vi "20.1.E122X.Group4.FinalExperimentAnalysis.vi"() -> ()   [LabVIEW 2014]
uses:
  <vilib>/Utility/miscctls.llb/LVDateTimeRec.ctl
  <vilib>/Analysis/baseanly.llb/Mean (DBL).vi
  <vilib>/Utility/file.llb/Read From Spreadsheet File (string).vi
  <vilib>/regexp/Match Regular Expression.xnode
  <vilib>/Analysis/NI_AALBase.lvlib
panel:
  in  "file path: CPU/GPU":path
  in  "file path: Environment":path
  in  "Tab Control":T1(tab)
  out "GPU":cluster{timestamp[], dbl[]}(graph)
  out "CPU":cluster{timestamp[], dbl[]}(graph)
  out "Humidity":cluster{timestamp[], dbl[]}(graph)
  out "Temperature":cluster{timestamp[], dbl[]}(graph)
  in  "Window Position":dbl(slide) min=3670814882.0 max=3671117162.0 scale=3670814882.0..3671117162.0 scale format="%<%I:%M %p\n%m/%d>T"
  in  "Window Size":dbl(slide) min=3670814882.0 max=3671117162.0 scale=240.0..302280.0 scale format="%<%H:%M>t"
  out "Light":cluster{timestamp[], dbl[]}(graph)
  out "Current Time":dbl format="%<%X\n%x>T"
  out "Light at index":dbl
  out "Humidity at index":dbl
  out "Temperature at index":dbl
  out "Light Max":dbl
  out "Humidity Max":dbl
  out "Temperature Max":dbl
  out "Light Min":dbl
  out "Humidity Min":dbl
  out "Temperature Min":dbl
  out "Light Average":dbl
  out "Humidity Average":dbl
  out "Temperature Average":dbl
  in  "Data Index":i64(slide) scale=0.0..2146.0
  out "Low Sun (1200-5000 lux)":bool
  out "Overcast day (700-1200 lux)":bool
  out "Bright room (50-700 lux)":bool
  out "Dark room (5-50 lux)":bool
  out "Moonlit night (.5-5 lux)":bool
  out "Dim Hallway (.01-.1 lux)":bool
  # "This section contains information to verify that the system is functional."
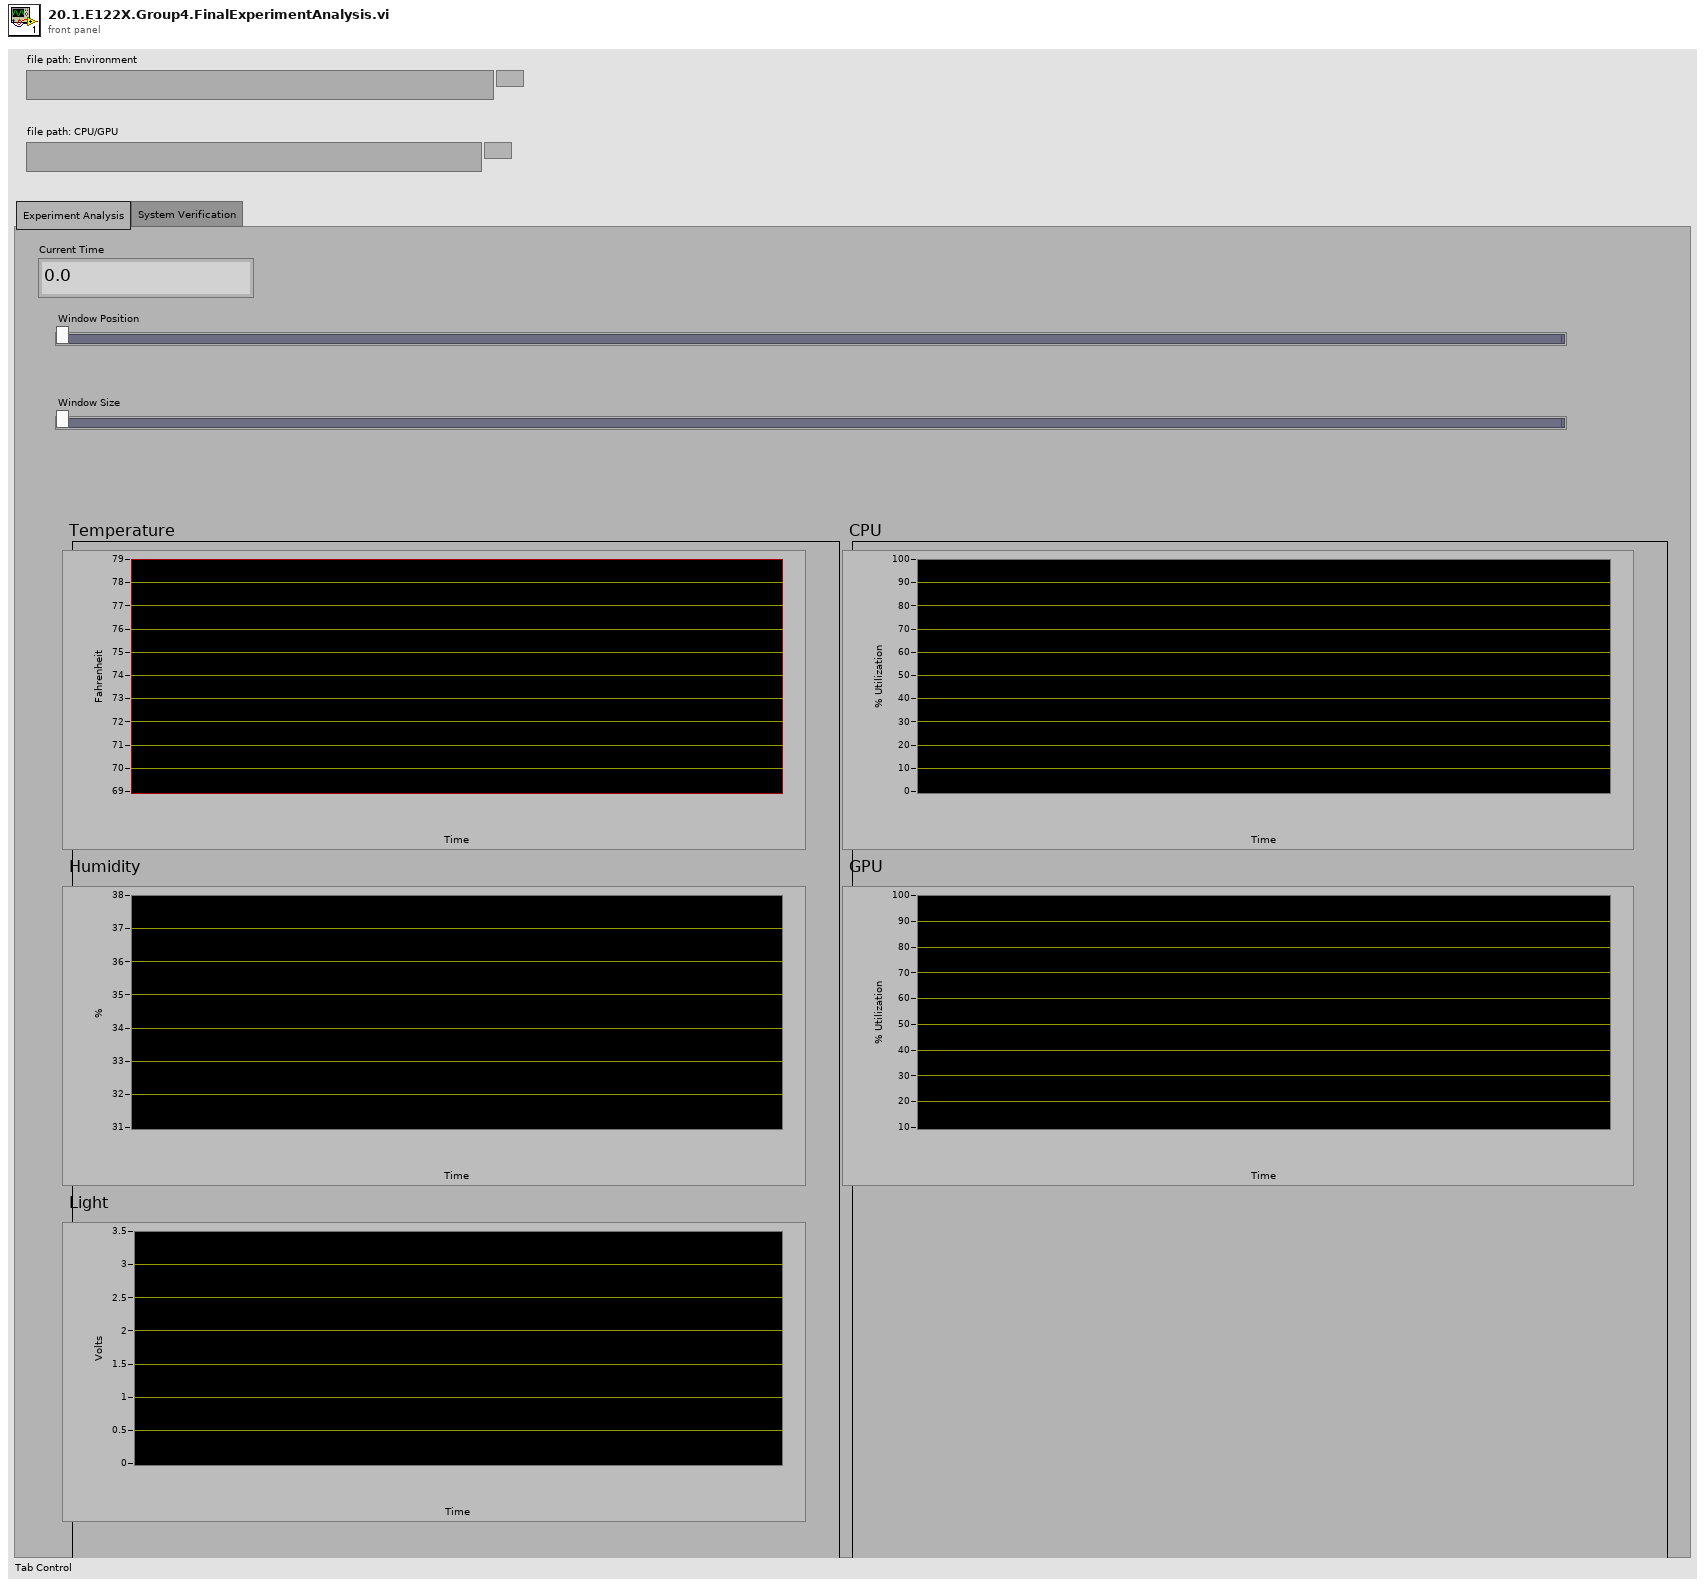
[diagram p1: front panel]
types:
  T1 = enum32{"Experiment Analysis", "System Verification"}
  T2 = typedef "LVDateTimeRec.ctl" = cluster{"fractional second":dbl, "second":i32, "minute":i32, "hour":i32, "day of month":i32, "month":i32, "year":i32, "day of week":i32, "day of year":i32, "DST":i32}
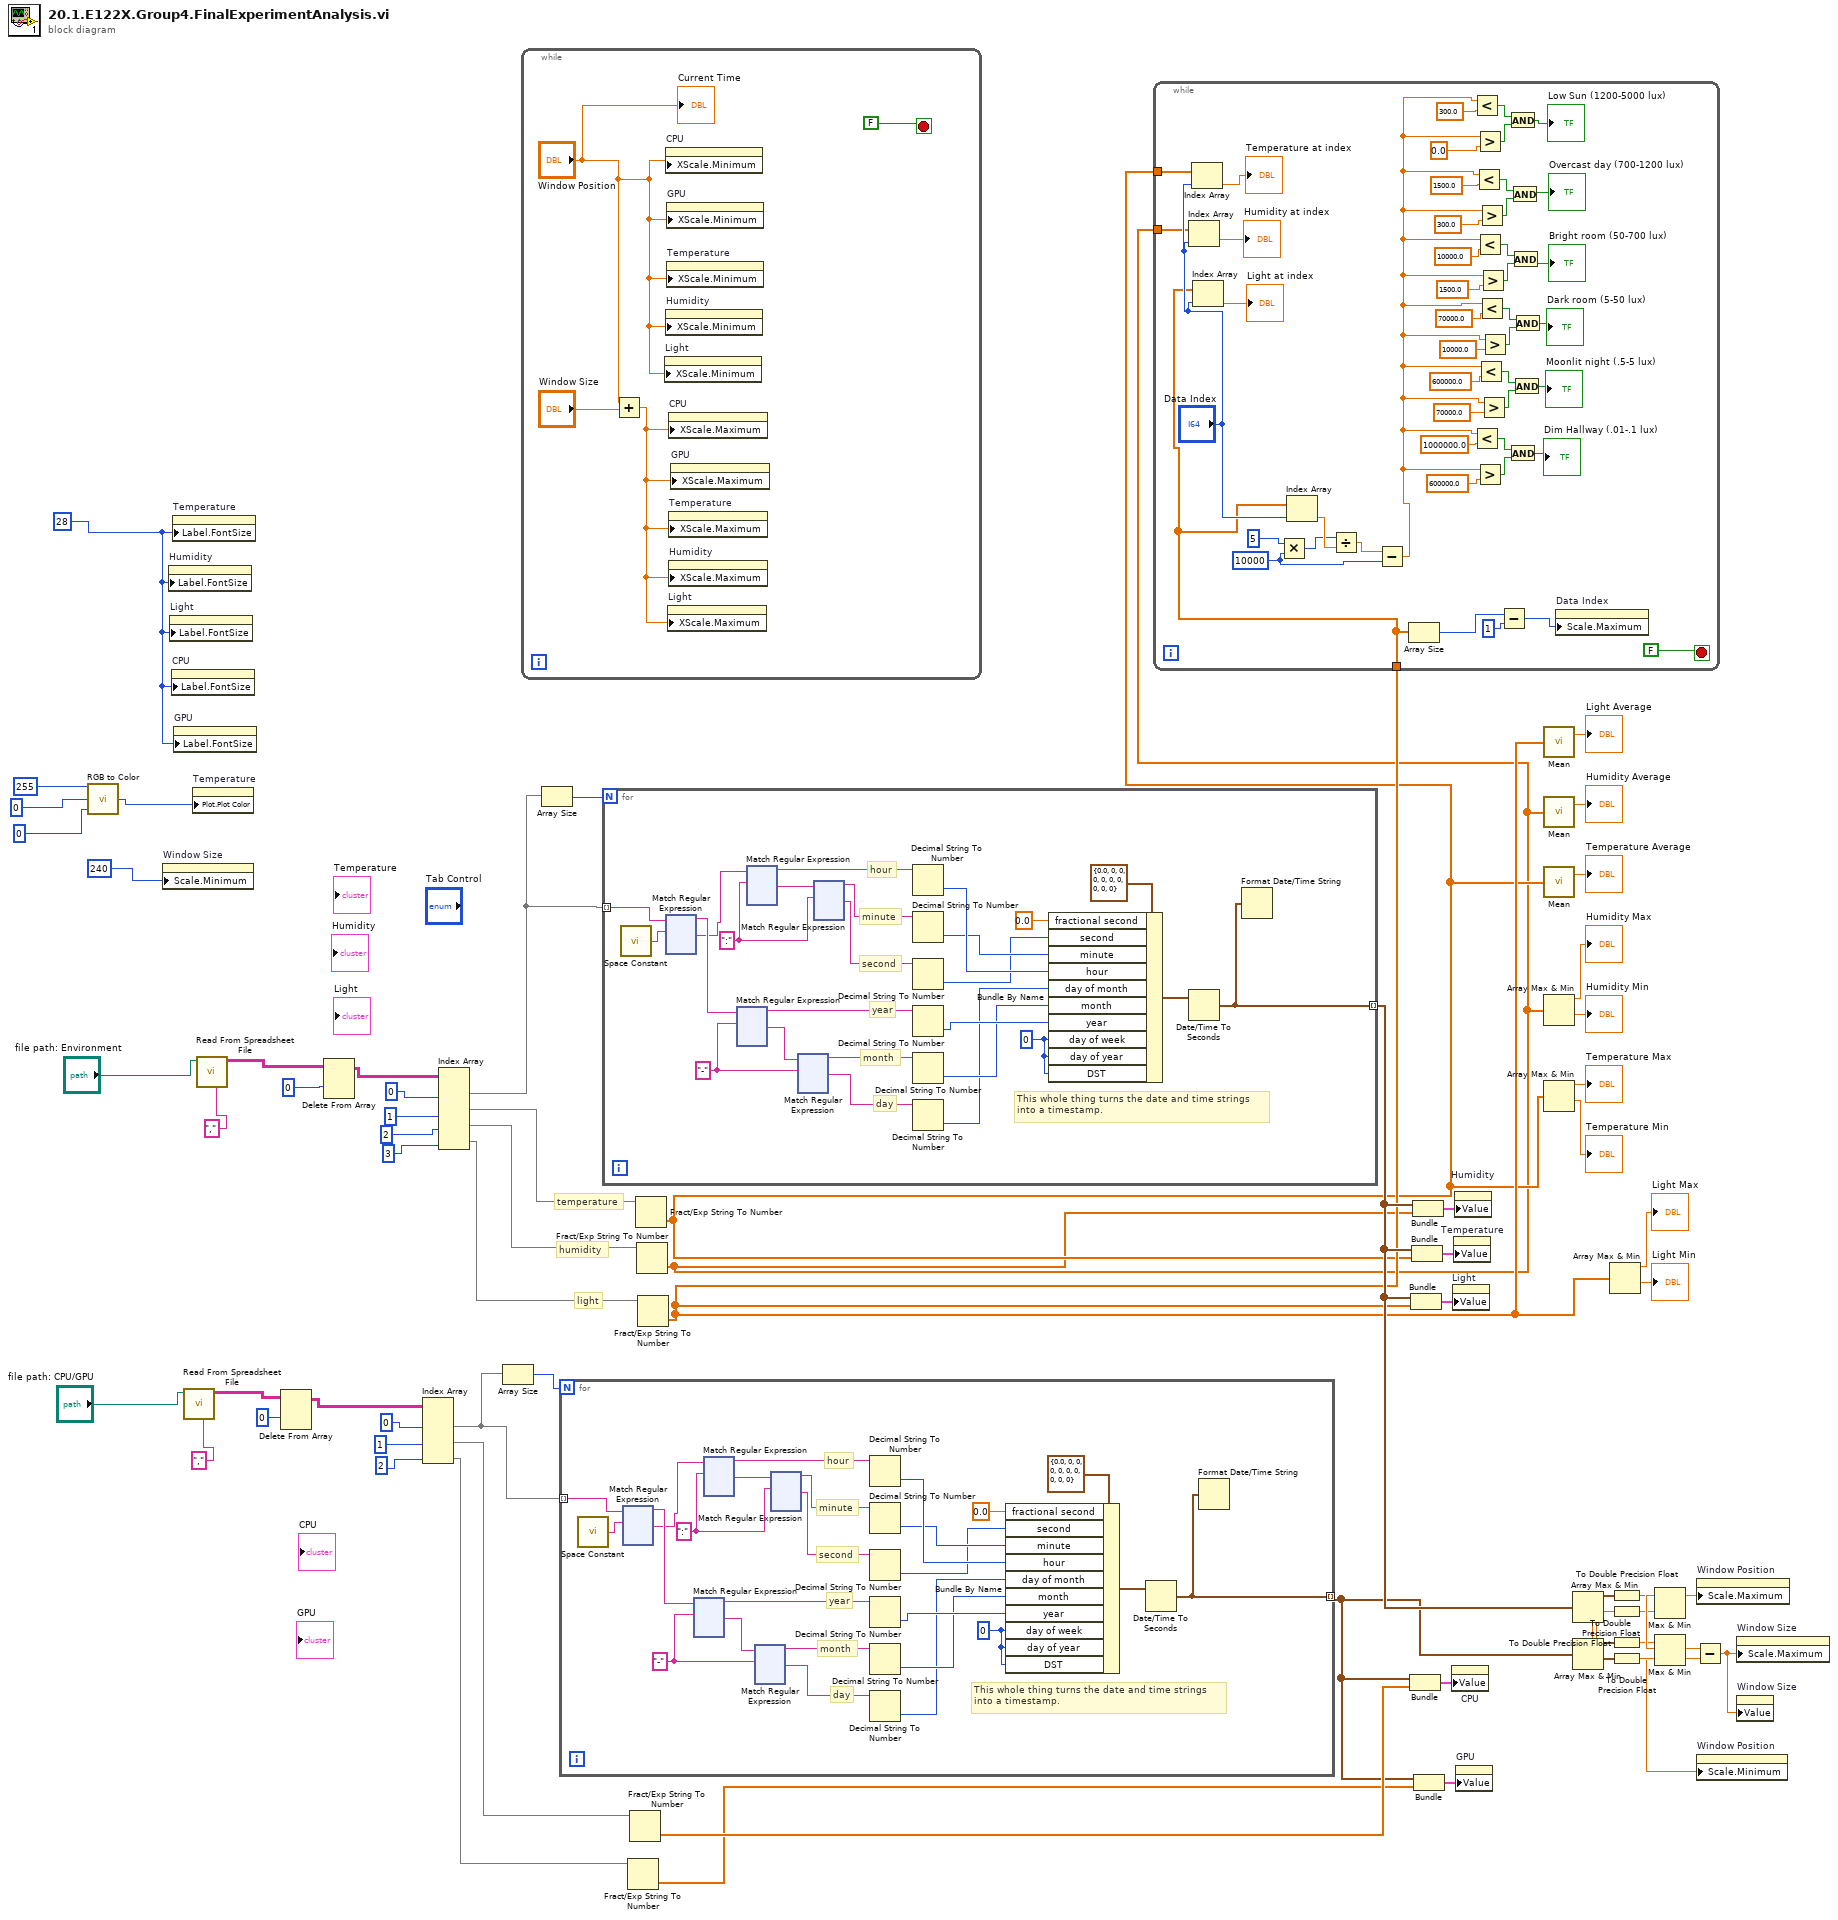
[diagram p0: block diagram]
diagram:
  w14 = 28
  # "light"
  # "humidity"
  # "temperature"
  n1 = call <vilib>:"RGB to Color.vi"("B"=0, "G"=0, "R"=255) -> ("Color"=w18:u32)
  n2 = property on="Window Size" class="Slide (strict)"("Scale.Minimum"=240) -> ()  [unwired: 2 in, 2 out]
  n3 = property on="Humidity" class="XYGraph (strict)"("Label.FontSize"=w14) -> ()  [unwired: 2 in, 2 out]
  n4 = property on="Light" class="XYGraph (strict)"("Label.FontSize"=w14) -> ()  [unwired: 2 in, 2 out]
  n5 = property on="CPU" class="XYGraph (strict)"("Label.FontSize"=w14) -> ()  [unwired: 2 in, 2 out]
  n6 = property on="Temperature" class="XYGraph (strict)"("Label.FontSize"=w14) -> ()  [unwired: 2 in, 2 out]
  n7 = property on="GPU" class="XYGraph (strict)"("Label.FontSize"=w14) -> ()  [unwired: 2 in, 2 out]
  n8 = call-poly <vilib>:"Read From Spreadsheet File.vi"("delimiter (\\t)"="," ("delimiter (\\t)"), "file path (dialog if empty)"="file path: CPU/GPU") -> ("all rows"=w54:string[][])  [unwired: 5 in, 4 out]
  n9 = property on="Temperature" class="XYGraph (strict)"("Plot.Plot Color"=w18) -> ()  [unwired: 2 in, 2 out]
  n10 = call-poly <vilib>:"Read From Spreadsheet File.vi"("delimiter (\\t)"="," ("delimiter (\\t)"), "file path (dialog if empty)"="file path: Environment") -> ("all rows"=w56:string[][])  [unwired: 5 in, 4 out]
  n11 = Delete From Array(array=w54, index (row)=0) -> (array with subset deleted=w46:string[][])  [unwired: 2 in, 1 out]
  n12 = Delete From Array(array=w56, index (row)=0) -> (array with subset deleted=w52:string[][])  [unwired: 2 in, 1 out]
  n13 = Index Array(array=w46, index (col) #1=0 ("disabled index (col)"), index (col) #2=1 ("disabled index (col)"), index (col) #3=2 ("disabled index (col)")) -> (element #1=w42:string[], element #2=w44:string[], element #3=w45:string[])  [unwired: 3 in]
  n14 = Index Array(array=w52, index (col) #1=0 ("disabled index (col)"), index (col) #2=1 ("index (col)"), index (col) #3=2 ("index (col)"), index (col) #4=3 ("index (col)")) -> (element #1=w50:string[], element #2=w49:string[], element #3=w48:string[], element #4=w47:string[])  [unwired: 4 in]
  n15 = Array Size(array=w42) -> (size(s)=w43:i32)
  n16 = while {
    stop <- FALSE stop-if-true
    n17 = Add(x="Window Position", y="Window Size") -> (x+y=w65:dbl)
    n18 = property on="Light" class="XYGraph (strict)"("XScale.Minimum"="Window Position") -> ()  [unwired: 2 in, 2 out]
    n19 = property on="CPU" class="XYGraph (strict)"("XScale.Minimum"="Window Position") -> ()  [unwired: 2 in, 2 out]
    n20 = property on="Humidity" class="XYGraph (strict)"("XScale.Minimum"="Window Position") -> ()  [unwired: 2 in, 2 out]
    n21 = property on="GPU" class="XYGraph (strict)"("XScale.Minimum"="Window Position") -> ()  [unwired: 2 in, 2 out]
    n22 = property on="Temperature" class="XYGraph (strict)"("XScale.Minimum"="Window Position") -> ()  [unwired: 2 in, 2 out]
    n23 = property on="Light" class="XYGraph (strict)"("XScale.Maximum"=w65) -> ()  [unwired: 2 in, 2 out]
    n24 = property on="CPU" class="XYGraph (strict)"("XScale.Maximum"=w65) -> ()  [unwired: 2 in, 2 out]
    n25 = property on="Temperature" class="XYGraph (strict)"("XScale.Maximum"=w65) -> ()  [unwired: 2 in, 2 out]
    n26 = property on="Humidity" class="XYGraph (strict)"("XScale.Maximum"=w65) -> ()  [unwired: 2 in, 2 out]
    n27 = property on="GPU" class="XYGraph (strict)"("XScale.Maximum"=w65) -> ()  [unwired: 2 in, 2 out]
    "Current Time" <- "Window Position"
  }
  n28 = Array Size(array=w50) -> (size(s)=w51:i32)
  n29 = for {
    N: w43 -> [_]
    tunnel: w42 -> [w75] mode=indexing
    tunnel: [w69] -> w13 mode=indexing
    w79 = 0 ("day of week")
    w76 = ":" ("regular expression")
    w93 = "-" ("regular expression")
    # "This whole thing turns the date and time strings\ninto a timestamp."
    # "second"
    # "minute"
    # "hour"
    # "year"
    # "day"
    # "month"
    n30 = call <vilib>:"Space Constant.vi"() -> ("String"=w77:string)
    n31 = xnode "Match Regular Expression"("input string"=w75, "regular expression"=w77) -> ("before match"=w71:string, "after match"=w70:string)  [unwired: 4 in, 3 out]
    n32 = xnode "Match Regular Expression"("input string"=w71, "regular expression"=w93) -> ("before match"=w90:string, "after match"=w92:string)  [unwired: 4 in, 3 out]
    n33 = xnode "Match Regular Expression"("input string"=w70, "regular expression"=w76) -> ("before match"=w87:string, "after match"=w91:string)  [unwired: 4 in, 3 out]
    n34 = xnode "Match Regular Expression"("input string"=w92, "regular expression"=w93) -> ("before match"=w89:string, "after match"=w88:string)  [unwired: 4 in, 3 out]
    n35 = xnode "Match Regular Expression"("input string"=w91, "regular expression"=w76) -> ("before match"=w86:string, "after match"=w85:string)  [unwired: 4 in, 3 out]
    n36 = Decimal String To Number(string=w87) -> (number=w83:i32)  [unwired: 2 in, 1 out]
    n37 = Decimal String To Number(string=w86) -> (number=w82:i32)  [unwired: 2 in, 1 out]
    n38 = Decimal String To Number(string=w85) -> (number=w81:i32)  [unwired: 2 in, 1 out]
    n39 = Decimal String To Number(string=w90) -> (number=w74:i32)  [unwired: 2 in, 1 out]
    n40 = Decimal String To Number(string=w89) -> (number=w73:i32)  [unwired: 2 in, 1 out]
    n41 = Decimal String To Number(string=w88) -> (number=w72:i32)  [unwired: 2 in, 1 out]
    n42 = Bundle By Name(cluster=T2 {"fractional second"=0.0, "second"=0, "minute"=0, "hour"=0, "day of month"=0, "month"=0, "year"=0, "day of week"=0, "day of year"=0, "DST"=0} ("date time rec"), "fractional second"=0.0, "second"=w81, "minute"=w82, "hour"=w83, "day of month"=w72, "month"=w73, "year"=w74, "day of week"=w79, "day of year"=w79, "DST"=w79) -> (w80:T2)
    n43 = Date/Time To Seconds(2:w80) -> (0:w69:timestamp)  [unwired: 1 in]
    n44 = Format Date/Time String(seconds (now)=w69) -> ()  [unwired: 2 in, 1 out]
  }
  n45 = for {
    N: w51 -> [_]
    tunnel: w50 -> [w670] mode=indexing
    tunnel: [w664] -> w24 mode=indexing
    w674 = 0 ("day of week")
    w671 = ":" ("regular expression")
    w688 = "-" ("regular expression")
    # "This whole thing turns the date and time strings\ninto a timestamp."
    # "second"
    # "minute"
    # "hour"
    # "year"
    # "day"
    # "month"
    n46 = call <vilib>:"Space Constant.vi"() -> ("String"=w672:string)
    n47 = xnode "Match Regular Expression"("input string"=w670, "regular expression"=w672) -> ("before match"=w666:string, "after match"=w665:string)  [unwired: 4 in, 3 out]
    n48 = xnode "Match Regular Expression"("input string"=w666, "regular expression"=w688) -> ("before match"=w685:string, "after match"=w687:string)  [unwired: 4 in, 3 out]
    n49 = xnode "Match Regular Expression"("input string"=w665, "regular expression"=w671) -> ("before match"=w682:string, "after match"=w686:string)  [unwired: 4 in, 3 out]
    n50 = xnode "Match Regular Expression"("input string"=w687, "regular expression"=w688) -> ("before match"=w684:string, "after match"=w683:string)  [unwired: 4 in, 3 out]
    n51 = xnode "Match Regular Expression"("input string"=w686, "regular expression"=w671) -> ("before match"=w681:string, "after match"=w680:string)  [unwired: 4 in, 3 out]
    n52 = Decimal String To Number(string=w682) -> (number=w678:i32)  [unwired: 2 in, 1 out]
    n53 = Decimal String To Number(string=w681) -> (number=w677:i32)  [unwired: 2 in, 1 out]
    n54 = Decimal String To Number(string=w680) -> (number=w676:i32)  [unwired: 2 in, 1 out]
    n55 = Decimal String To Number(string=w685) -> (number=w669:i32)  [unwired: 2 in, 1 out]
    n56 = Decimal String To Number(string=w684) -> (number=w668:i32)  [unwired: 2 in, 1 out]
    n57 = Decimal String To Number(string=w683) -> (number=w667:i32)  [unwired: 2 in, 1 out]
    n58 = Bundle By Name(cluster=T2 {"fractional second"=0.0, "second"=0, "minute"=0, "hour"=0, "day of month"=0, "month"=0, "year"=0, "day of week"=0, "day of year"=0, "DST"=0} ("date time rec"), "fractional second"=0.0, "second"=w676, "minute"=w677, "hour"=w678, "day of month"=w667, "month"=w668, "year"=w669, "day of week"=w674, "day of year"=w674, "DST"=w674) -> (w675:T2)
    n59 = Date/Time To Seconds(2:w675) -> (0:w664:timestamp)  [unwired: 1 in]
    n60 = Format Date/Time String(seconds (now)=w664) -> ()  [unwired: 2 in, 1 out]
  }
  n61 = Fract/Exp String To Number(string=w45) -> (number=w36:dbl[])  [unwired: 3 in, 1 out]
  n62 = Fract/Exp String To Number(string=w44) -> (number=w38:dbl[])  [unwired: 3 in, 1 out]
  n63 = Fract/Exp String To Number(string=w49) -> (number=w2:dbl[])  [unwired: 3 in, 1 out]
  n64 = Fract/Exp String To Number(string=w48) -> (number=w1:dbl[])  [unwired: 3 in, 1 out]
  n65 = Fract/Exp String To Number(string=w47) -> (number=w3:dbl[])  [unwired: 3 in, 1 out]
  n66 = while {
    tunnel: w3 -> [w1259]
    tunnel: w2 -> [w1261]
    tunnel: w1 -> [w1260]
    stop <- FALSE stop-if-true
    w1269 = 10000
    n67 = Index Array(array=w1260, index="Data Index") -> (element=→"Humidity at index":dbl)
    n68 = Index Array(array=w1261, index="Data Index") -> (element=→"Temperature at index":dbl)
    n69 = Index Array(array=w1259, index="Data Index") -> (element=→"Light at index":dbl)
    n70 = Multiply(x=5, y=w1269) -> (x*y=w1271:i32)
    n71 = Index Array(array=w1259, index="Data Index") -> (element=w1272:dbl)
    n72 = Divide(x=w1271, y=w1272) -> (x/y=w1274:dbl)
    n73 = Subtract(x=w1274, y=w1269) -> (x-y=w1273:dbl)
    n74 = Array Size(array=w1259) -> (size(s)=w1268:i32)
    n75 = Less?(x=w1273, y=300.0) -> (x < y?=w1301:bool)
    n76 = Less?(x=w1273, y=1000000.0) -> (x < y?=w1277:bool)
    n77 = Less?(x=w1273, y=1500.0) -> (x < y?=w1296:bool)
    n78 = Greater?(x=w1273, y=0.0) -> (0:w1302:bool)
    n79 = Less?(x=w1273, y=10000.0) -> (x < y?=w1291:bool)
    n80 = Greater?(x=w1273, y=600000.0) -> (0:w1278:bool)
    n81 = Less?(x=w1273, y=600000.0) -> (x < y?=w1281:bool)
    n82 = Greater?(x=w1273, y=300.0) -> (0:w1297:bool)
    n83 = Less?(x=w1273, y=70000.0) -> (x < y?=w1285:bool)
    n84 = Greater?(x=w1273, y=1500.0) -> (0:w1292:bool)
    n85 = Greater?(x=w1273, y=70000.0) -> (0:w1282:bool)
    n86 = Greater?(x=w1273, y=10000.0) -> (0:w1286:bool)
    n87 = Subtract(x=w1268, y=1) -> (x-y=w1267:i32)
    n88 = And(x=w1301, y=w1302) -> (x .and. y?=→"Low Sun (1200-5000 lux)":bool)
    n89 = And(x=w1277, y=w1278) -> (x .and. y?=→"Dim Hallway (.01-.1 lux)":bool)
    n90 = And(x=w1296, y=w1297) -> (x .and. y?=→"Overcast day (700-1200 lux)":bool)
    n91 = And(x=w1291, y=w1292) -> (x .and. y?=→"Bright room (50-700 lux)":bool)
    n92 = And(x=w1281, y=w1282) -> (x .and. y?=→"Moonlit night (.5-5 lux)":bool)
    n93 = And(x=w1285, y=w1286) -> (x .and. y?=→"Dark room (5-50 lux)":bool)
    n94 = property on="Data Index" class="Slide (strict)"("Scale.Maximum"=w1267) -> ()  [unwired: 2 in, 2 out]
  }
  n95 = Bundle(w13, w38) -> (w37:cluster{timestamp[], dbl[]})  [unwired: 1 in]
  n96 = Bundle(w24, w3) -> (w34:cluster{timestamp[], dbl[]})  [unwired: 1 in]
  n97 = Bundle(w24, w2) -> (w32:cluster{timestamp[], dbl[]})  [unwired: 1 in]
  n98 = Bundle(w24, w1) -> (w33:cluster{timestamp[], dbl[]})  [unwired: 1 in]
  n99 = Bundle(w13, w36) -> (w35:cluster{timestamp[], dbl[]})  [unwired: 1 in]
  n100 = property on="CPU" class="XYGraph (strict)"("Value"=w37) -> ()  [unwired: 2 in, 2 out]
  n101 = property on="Light" class="XYGraph (strict)"("Value"=w34) -> ()  [unwired: 2 in, 2 out]
  n102 = property on="Temperature" class="XYGraph (strict)"("Value"=w32) -> ()  [unwired: 2 in, 2 out]
  n103 = property on="Humidity" class="XYGraph (strict)"("Value"=w33) -> ()  [unwired: 2 in, 2 out]
  n104 = property on="GPU" class="XYGraph (strict)"("Value"=w35) -> ()  [unwired: 2 in, 2 out]
  n105 = call-poly <vilib>:"Mean.vi"("X"=w3) -> ("mean"=→"Light Average":dbl)  [unwired: 1 out]
  n106 = call-poly <vilib>:"Mean.vi"("X"=w1) -> ("mean"=→"Humidity Average":dbl)  [unwired: 1 out]
  n107 = call-poly <vilib>:"Mean.vi"("X"=w2) -> ("mean"=→"Temperature Average":dbl)  [unwired: 1 out]
  n108 = Array Max & Min(array=w1) -> (max value=→"Humidity Max":dbl, min value=→"Humidity Min":dbl)  [unwired: 2 out]
  n109 = Array Max & Min(array=w2) -> (max value=→"Temperature Max":dbl, min value=→"Temperature Min":dbl)  [unwired: 2 out]
  n110 = Array Max & Min(array=w24) -> (max value=w23:timestamp, min value=w22:timestamp)  [unwired: 2 out]
  n111 = Array Max & Min(array=w13) -> (max value=w31:timestamp, min value=w30:timestamp)  [unwired: 2 out]
  n112 = Array Max & Min(array=w3) -> (max value=→"Light Max":dbl, min value=→"Light Min":dbl)  [unwired: 2 out]
  n113 = To Double Precision Float(number=w23) -> (double precision float=w20:dbl)
  n114 = To Double Precision Float(number=w22) -> (double precision float=w21:dbl)
  n115 = To Double Precision Float(number=w31) -> (double precision float=w25:dbl)
  n116 = To Double Precision Float(number=w30) -> (double precision float=w26:dbl)
  n117 = Max & Min(x=w20, y=w25) -> (max(x,y)=w27:dbl)  [unwired: 1 out]
  n118 = Max & Min(x=w21, y=w26) -> (min(x,y)=w19:dbl)  [unwired: 1 out]
  n119 = Subtract(x=w27, y=w19) -> (x-y=w28:dbl)
  n120 = property on="Window Position" class="Slide (strict)"("Scale.Maximum"=w27) -> ()  [unwired: 2 in, 2 out]
  n121 = property on="Window Position" class="Slide (strict)"("Scale.Minimum"=w19) -> ()  [unwired: 2 in, 2 out]
  n122 = property on="Window Size" class="Slide (strict)"("Scale.Maximum"=w28) -> ()  [unwired: 2 in, 2 out]
  n123 = property on="Window Size" class="Slide (strict)"("Value"=w28) -> ()  [unwired: 2 in, 2 out]
